vi "Enqueue Data.vi"(8 "error in (no error)":errorcluster, 10 "Data":dbl, 11 "Test 1 API in":refnum<class "Test 1 API.lvclass">) -> (0 "error out":errorcluster, 3 "Test 1 API out":refnum<class "Test 1 API.lvclass">)   [LabVIEW 2020, in "Scratchpad.lvlib" / "Test 1.lvlib" / "Test 1 API.lvclass"]
uses:
  Test 1 API.lvclass
  Artifex/Actor Proxy/Actor API.lvclass
  Enqueue Data Msg/Enqueue Data Msg.lvclass
  Artifex/Priority.ctl
  Artifex/Artifex.lvlib
panel:
  in  "Priority (Normal)":T1=enum."Normal"
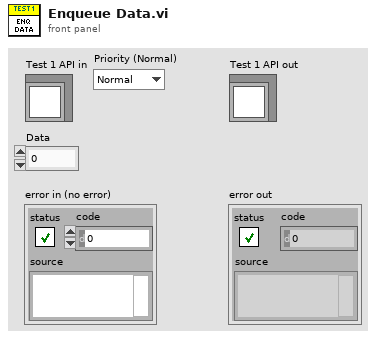
[diagram p1: front panel]
types:
  T1 = typedef "Artifex.lvlib/Priority.ctl" = enum16{"Low", "Normal", "High"}
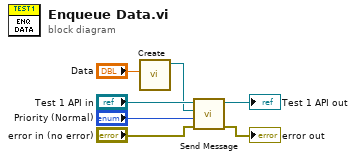
[diagram p0: block diagram]
diagram:
  n1 = call "Create.vi"("Data"="Data") -> ("Enqueue Data Msg out"=w1:refnum<class "Enqueue Data Msg.lvclass">)  [unwired: 9 in, 1 out]
  n2 = call "Send Message.vi"("error in (no error)"="error in (no error)", "Priority (Normal)"="Priority (Normal)", "Message"=w1, "Actor API in"="Test 1 API in") -> ("error out"=→"error out":errorcluster, "Actor API out"=→"Test 1 API out":refnum<class "Test 1 API.lvclass">)  [unwired: 6 in]
